vi "SQL Time to Timestamp.vi"(1 "date/time string":string) -> (0 "Time Stamp":timestamp)   [LabVIEW 2019, in "LV-Data.PGSQL.lvclass"]
uses:
  LV-Data.PGSQL.lvclass
panel:
  out "error out":errorcluster
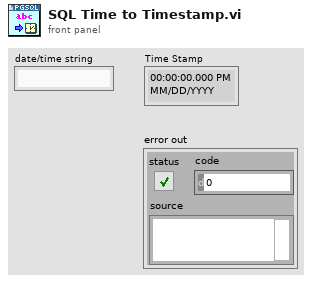
[diagram p1: front panel]
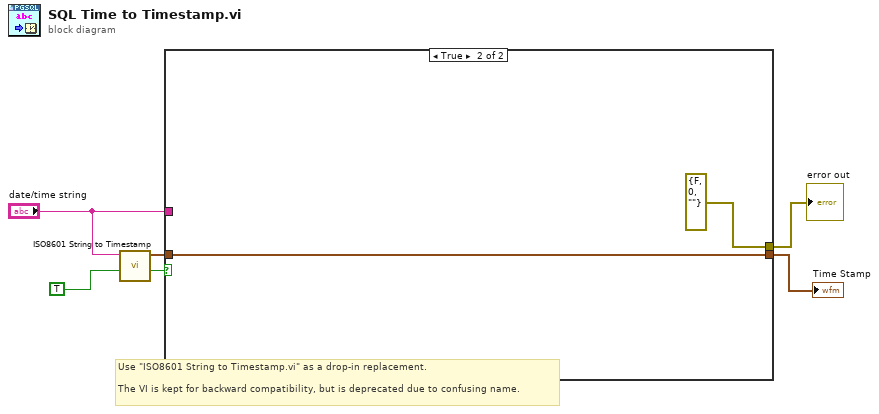
[diagram p0: block diagram]
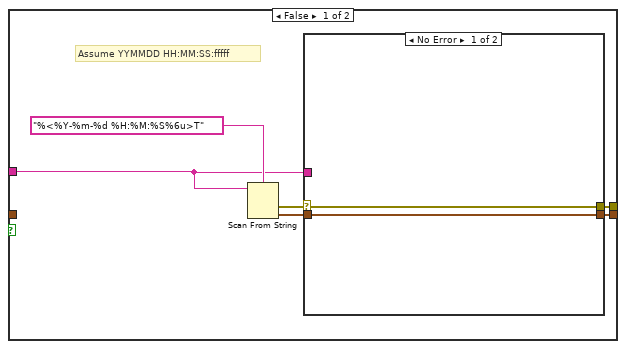
[diagram p2: hidden frame]
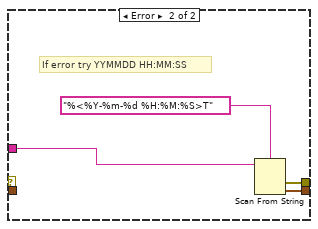
[diagram p3: hidden frame]
diagram:
  # "Use \"ISO8601 String to Timestamp.vi\" as a drop-in replacement.\n\nThe VI is kept for backward compatibility, but is deprecated due to confusing name."
  n1 = call <vilib>:"ISO8601 String to Timestamp.vi"("Strict ISO? (T)"=TRUE, "ISO8601 String"="date/time string") -> ("valid?"=w3:bool, "Timestamp"=w2:timestamp)  [unwired: 7 in, 1 out]
  n2 = case shown="True" w3 {
    tunnel: [w9 errorcluster {"status"=FALSE, "code"=0, "source"=""} ("error IO")] -> w6
    tunnel: [w8 w20] -> w5
    tunnel: "date/time string" -> [w7 _]
    tunnel: w2 -> [_ w20]
    frame False {
      # "Assume YYMMDD HH:MM:SS:fffff"
      n3 = Scan From String(format string="%<%Y-%m-%d %H:%M:%S%6u>T", input string=w7) -> (error out=w10:errorcluster, output 1=w12:timestamp)  [unwired: 3 in, 2 out]
      n4 = case shown="No Error" w10 {
        selector: w10 -> [w13 _]
        tunnel: w12 -> [w14 _]
        tunnel: [w14 w15] -> w8
        tunnel: [w13 w17] -> w9
        tunnel: w7 -> [_ w16]
        frame No Error {
        }
        frame Error {
          # "If error try YYMMDD HH:MM:SS"
          n5 = Scan From String(format string="%<%Y-%m-%d %H:%M:%S>T", input string=w16) -> (error out=w17:errorcluster, output 1=w15:timestamp)  [unwired: 3 in, 2 out]
        }
      }
    }
    frame True {
    }
  }
  "Time Stamp" <- w5
  "error out" <- w6
